vi "GetType.vi"(8 "error in (no error)":errorcluster, 11 "Configure Burst Count [BST] Msg":refnum<class "Configure Burst Count [BST] Msg.lvclass">) -> (0 "error out":errorcluster, 2 "Data Sample":variant, 3 "Configure Burst Count [BST] Msg":refnum<class "Configure Burst Count [BST] Msg.lvclass">)   [LabVIEW 2015, in "CS++Fgen.lvlib" / "Configure Burst Count [BST] Msg.lvclass"]
doc: "This VI delivers a sample of the data type format the message expects."
uses:
  Configure Burst Count [BST] Msg.lvclass
  Configure Burst Count [BST] Msg.lvclass/Configure Burst Count [BST] Msg.ctl
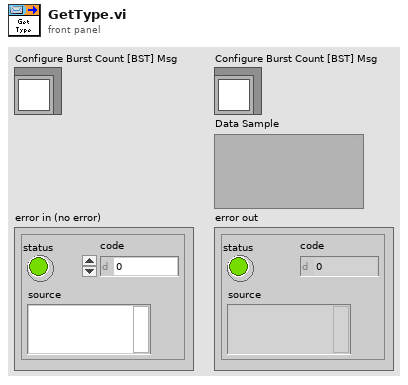
[diagram p1: front panel]
types:
  T1 = cluster{"Channel Name (\"\")":string, "burst count (1)":i32}
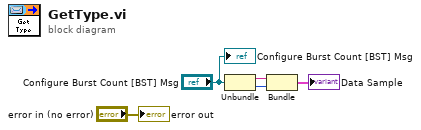
[diagram p0: block diagram]
diagram:
  n1 = Unbundle("Configure Burst Count [BST] Msg") -> (w2:string, w1:i32)
  n2 = Bundle("Channel Name (\"\")"=w2, "burst count (1)"=w1) -> (→"Data Sample":T1)  [unwired: 1 in]
  "error out" <- "error in (no error)"
  "Configure Burst Count [BST] Msg" <- "Configure Burst Count [BST] Msg"
